vi "DVR Q Loop.vi"(10 "DVR":refnum<data-value>) -> ()   [LabVIEW 2021, in "Q Async.lvlib"]
uses:
  Q Async.lvlib
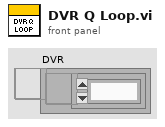
[diagram p1: front panel]
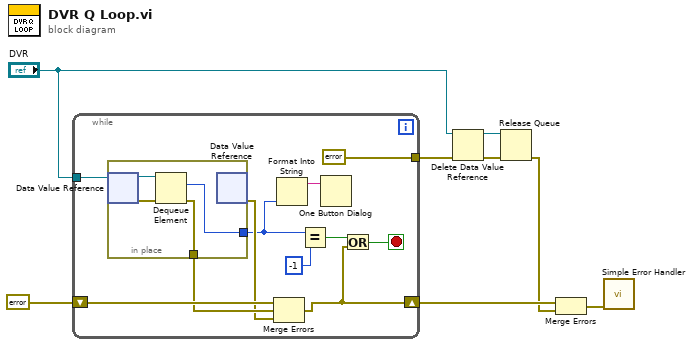
[diagram p0: block diagram]
diagram:
  n1 = while {
    tunnel: "DVR" -> [w17]
    shift-right: [w9] -> w6
    shift-left: errorcluster {"status"=FALSE, "code"=0, "source"=""} ("error IO") -> [w16]
    tunnel: [errorcluster {"status"=FALSE, "code"=0, "source"=""} ("error in (no error)")] -> w2
    stop <- w10 stop-if-true
    n2 = in-place {
      in-place-border: [w23] -> w12
      in-place-border: [w20] -> w15
      n3 = in-place-dvr #1(w17) -> (w22:refnum<queue>, w21:errorcluster)
      n4 = Dequeue Element(queue=w22, error in (no error)=w21) -> (element=w23:i32, error out=w20:errorcluster)  [unwired: 1 in, 2 out]
      n5 = in-place-dvr #1() -> (w14:errorcluster)  [unwired: 1 in, 1 out]
    }
    n6 = Merge Errors(w16, w15, w14) -> (w9:errorcluster)
    n7 = Format Into String(w12) -> (resulting string=w13:string)  [unwired: 3 in, 1 out]
    n8 = Equal?(x=w12, y=-1) -> (x = y?=w19:bool)
    n9 = One Button Dialog(message=w13) -> ()  [unwired: 1 in, 1 out]
    n10 = Or(x=w19, y=w9) -> (x .or. y?=w10:bool)
  }
  n11 = Delete Data Value Reference(data value reference="DVR", error in=w2) -> (data value=w7:refnum<queue>, error out=w3:errorcluster)
  n12 = Release Queue(queue=w7, error in (no error)=w3) -> (error out=w4:errorcluster)  [unwired: 1 in, 2 out]
  n13 = Merge Errors(w6, w4) -> (w5:errorcluster)
  n14 = call <vilib>:"Simple Error Handler.vi"("error in (no error)"=w5) -> ()  [unwired: 4 in, 5 out]
